vi "myRIO_BRig_Host_v0,21.vi"() -> ()   [LabVIEW 2014]
panel:
  out "graph":i32(graph)
  out "output_strAccum":string
  out "output_iTrial":i32
  out "BlockL_T2R_cur":u16 caption="Trials2Reward"
  out "BlockL_BTPR_cur":u16 caption="BadTrialsPostReward"
  out "BlockL_T2R_avg":dbl caption="Trials2Reward" format="%#_3g"
  out "BlockL_BTPR_avg":dbl caption="BadTrialsPostReward" format="%#_3g"
  out "BlockR_T2R_cur":u16 caption="Trials2Reward"
  out "BlockR_BTPR_cur":u16 caption="BadTrialsPostReward"
  out "BlockR_T2R_avg":dbl caption="Trials2Reward" format="%#_3g"
  out "BlockR_BTPR_avg":dbl caption="BadTrialsPostReward" format="%#_3g"
  out "RunTime_minutes":u16
  out "RunTime_seconds":u16
  out "error out 2":errorcluster caption="error out"
  in  "dataIn_maxTrialsDisplayed":u16 caption="Number of Trials Displayed\n( 0 = all trials )"
  in  "colorIn_timeout":u32(colorbox)=7468543 caption="Choice Timeout"
  in  "colorIn_wrong/cue":u32(colorbox)=16728618 caption="Wrong Choice or\nLicked During Cue"
  in  "colorIn_reward":u32(colorbox)=5898088 caption="Reward"
  in  "colorIn_unknown":u32(colorbox)=16449331 caption="Unknown Trial Status"
  in  "LoadPrevSettings":bool
  out "dataOut_plot":cluster{i32[], i32[]}[](graph)
  out "iBlock":u16
  out "iTrial":u16
  in  "stop":bool
  # "Exp Stats"
  # "Current Block Stats"
  # "Trials 2 Reward\n\nBad Trials\nPost Reward"
  # "Left Spout    Right Spout"
  # "Run Time\n\n   minutes    seconds"
  # "Average Block Stats"
  # "Trials 2 Reward\n\nBad Trials\nPost Reward"
  # "Left Spout    Right Spout"
  # "If you get ERROR 5 related to opening a file, press CONTINUE"
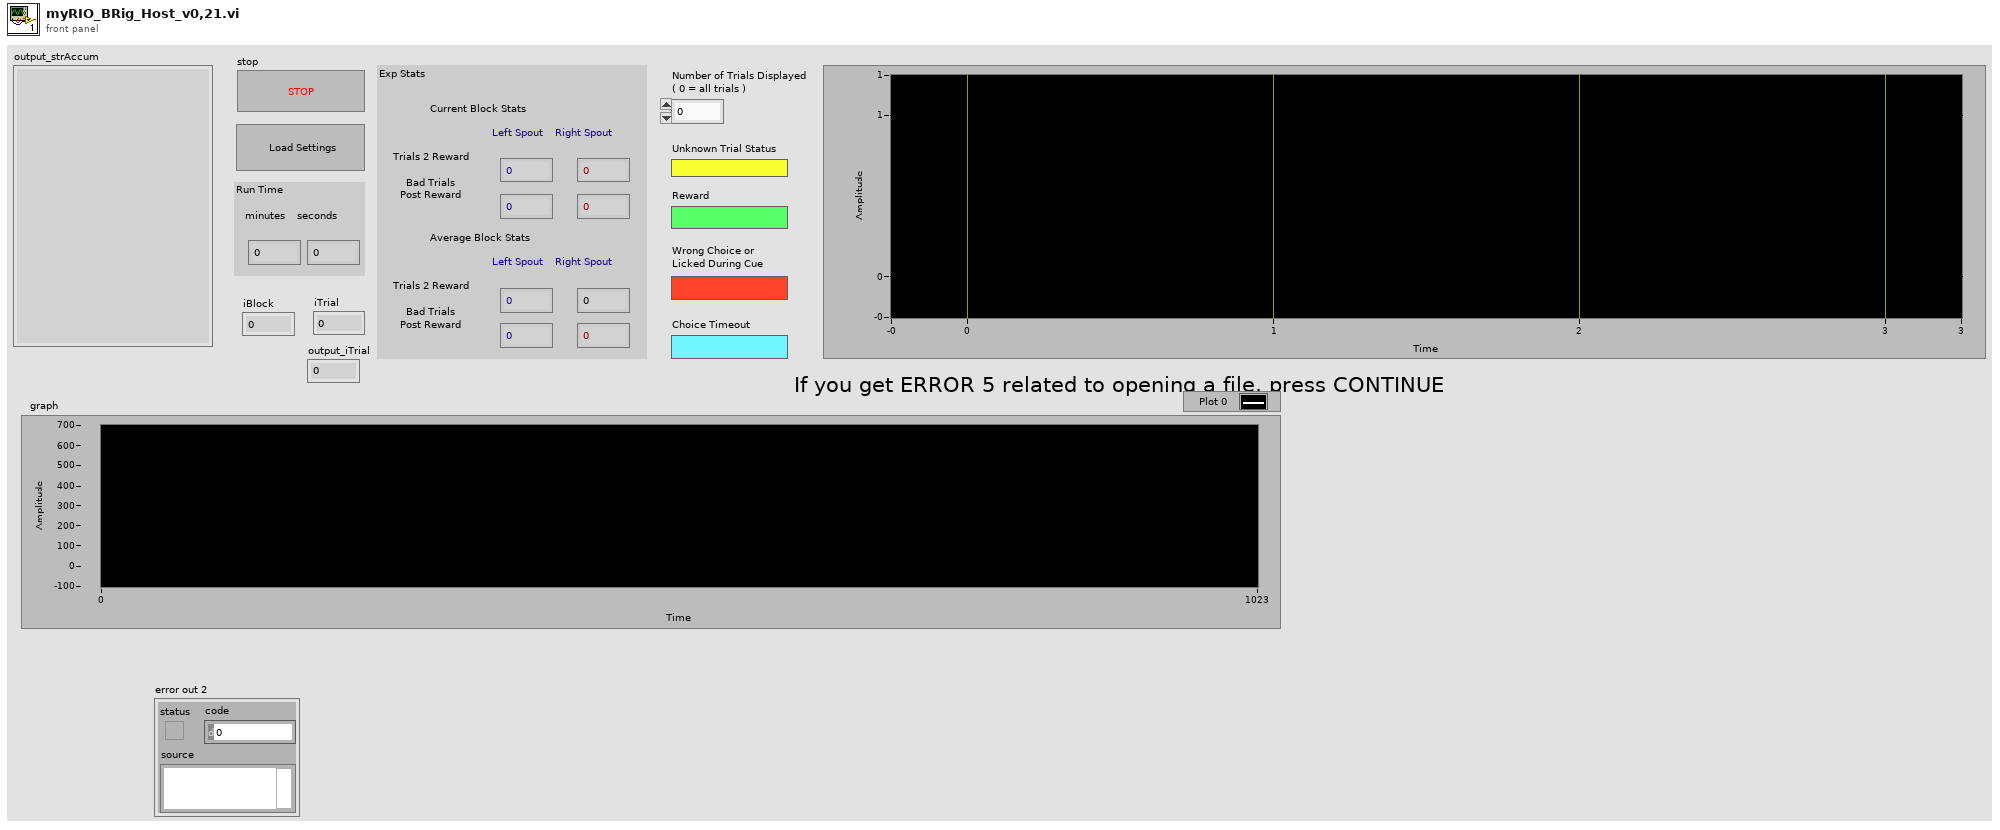
[diagram p1: front panel]
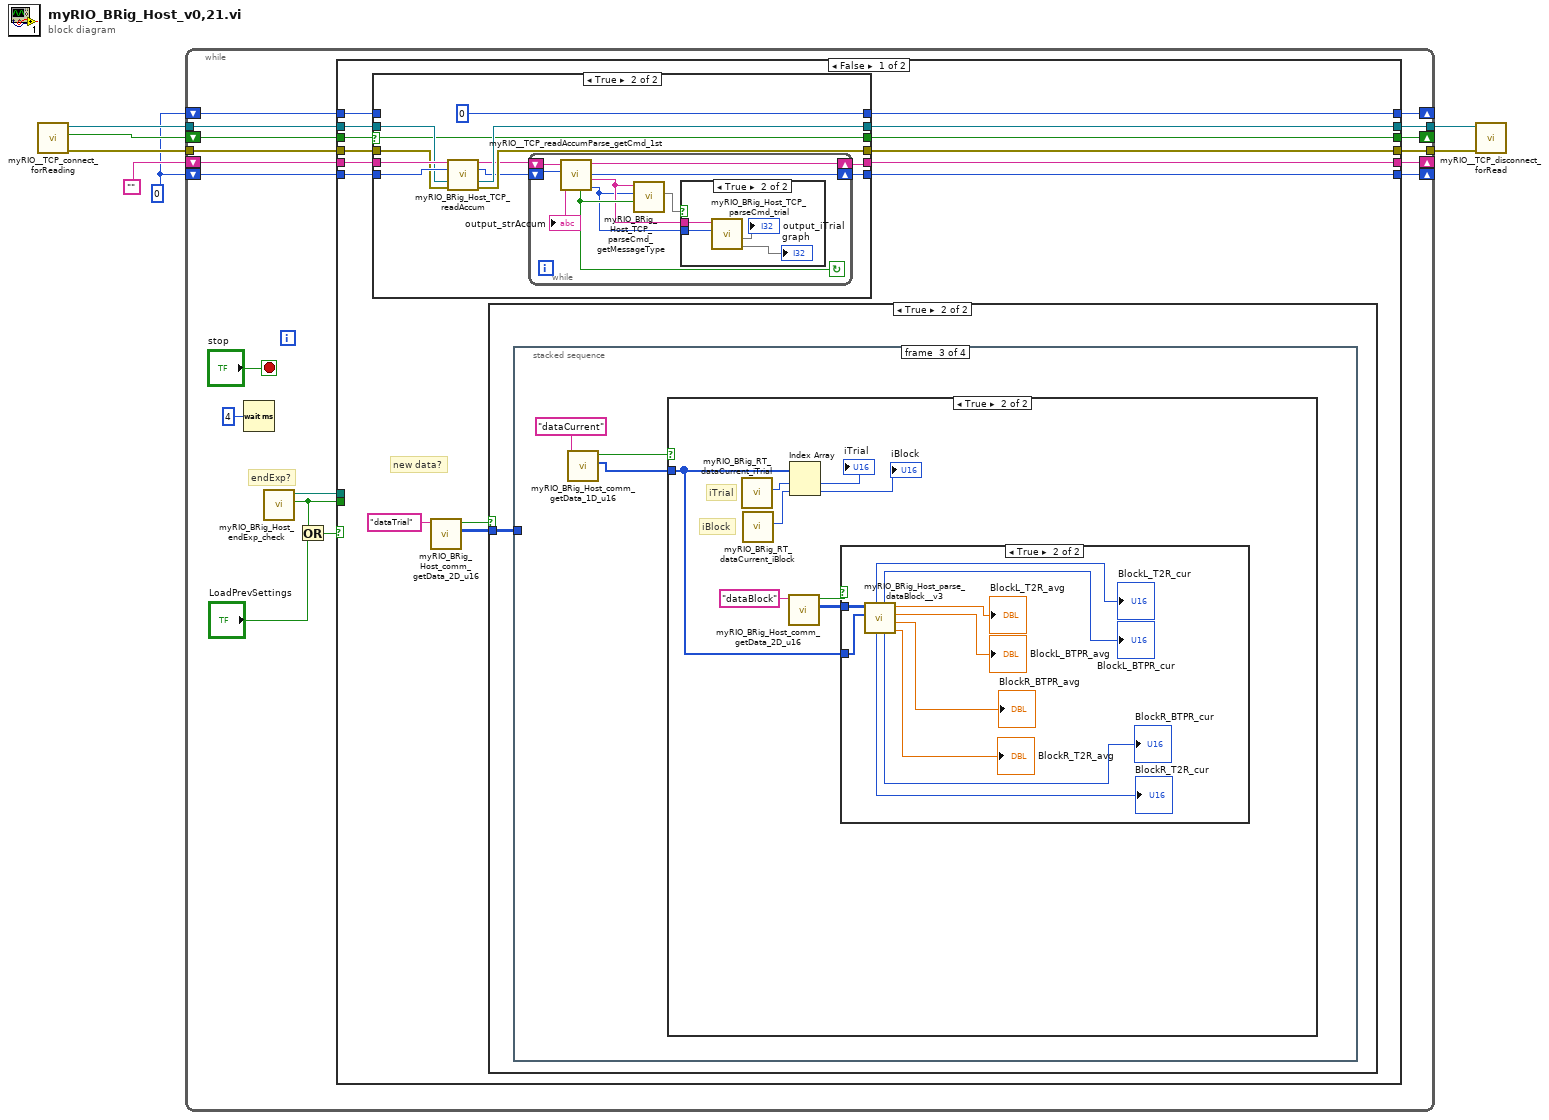
[diagram p0: block diagram]
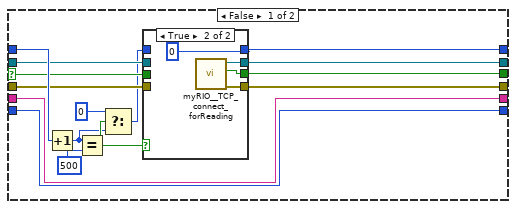
[diagram p2: hidden frame]
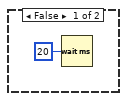
[diagram p5: hidden frame]
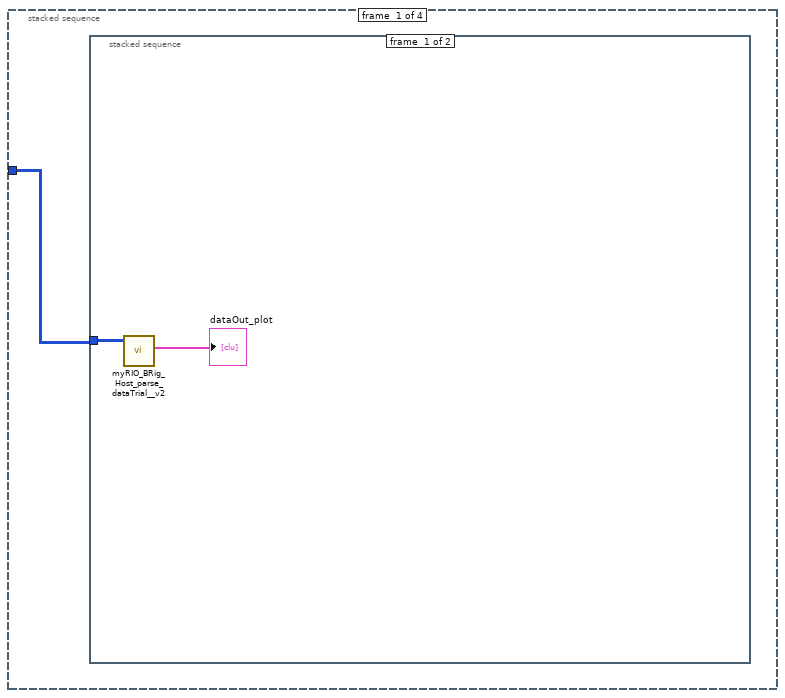
[diagram p6: hidden frame]
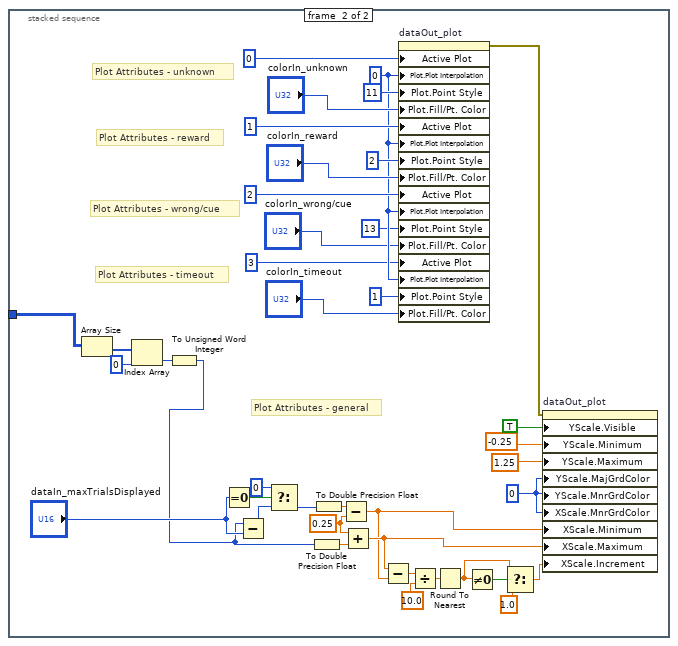
[diagram p7: hidden frame]
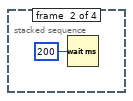
[diagram p8: hidden frame]
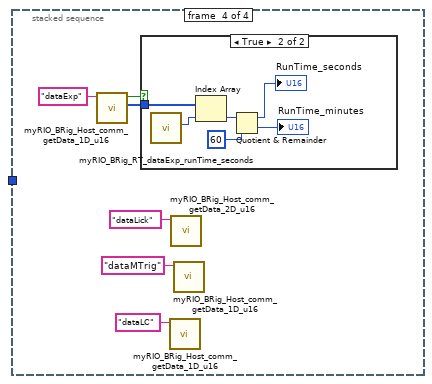
[diagram p11: hidden frame]
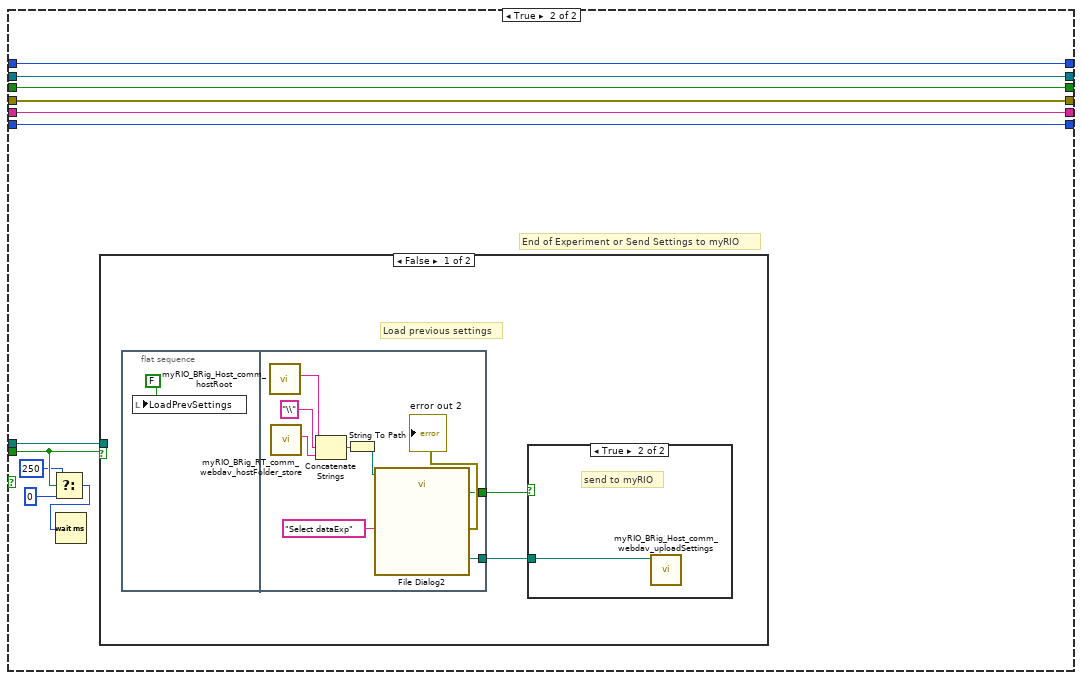
[diagram p13: hidden frame]
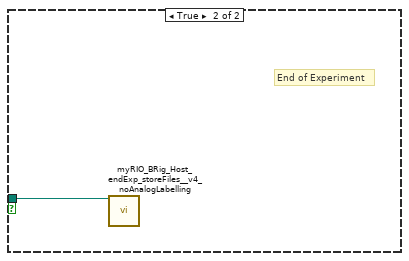
[diagram p15: hidden frame]
diagram:
  w1 = 0
  n1 = call "myRIO__TCP_connect_forReading.vi"() -> ("output_error"=w6:errorcluster, "output_connected"=w5:bool, "output_hTCP"=w7:refnum<k5>)  [unwired: 9 in]
  n2 = while {
    tunnel: w7 -> [w19]
    tunnel: w6 -> [w17]
    tunnel: [w18] -> w4
    tunnel: [w16] -> w3
    shift-right: [w13] -> _
    shift-left: "" -> [w15]
    shift-right: [w12] -> _
    shift-left: w1 -> [w14]
    shift-right: [w10] -> _
    shift-left: w5 -> [w11]
    shift-right: [w8] -> _
    shift-left: w1 -> [w9]
    stop <- "stop" stop-if-true
    # "endExp?"
    n3 = Wait (ms)(milliseconds to wait=u32 4) -> ()  [unwired: 1 out]
    n4 = call "myRIO_BRig_Host_endExp_check.vi"() -> ("output_IendExp"=w23:bool, "output_filePath_expExp"=w22:path)  [unwired: 10 in]
    n5 = Or(x=w23, y="LoadPrevSettings") -> (x .or. y?=w24:bool)
    n6 = case shown="False" w24 {
      tunnel: w23 -> [_ w176]
      tunnel: w22 -> [_ w177]
      tunnel: w19 -> [w33 w172]
      tunnel: [w32 w172] -> w18
      tunnel: w17 -> [w31 w171]
      tunnel: [w30 w171] -> w16
      tunnel: w15 -> [w37 w170]
      tunnel: w14 -> [w36 w169]
      tunnel: [w35 w170] -> w13
      tunnel: [w34 w169] -> w12
      tunnel: w11 -> [w29 w168]
      tunnel: [w28 w168] -> w10
      tunnel: w9 -> [w27 w167]
      tunnel: [w26 w167] -> w8
      frame False {
        # "new data?"
        n7 = case shown="True" w29 {
          selector: w29 -> [w48 w69]
          tunnel: w37 -> [w41 w75]
          tunnel: w36 -> [w42 w74]
          tunnel: [w41 w65] -> w35
          tunnel: [w42 w64] -> w34
          tunnel: w33 -> [w49 w73]
          tunnel: [w52 w72] -> w32
          tunnel: w31 -> [w47 w71]
          tunnel: [w51 w70] -> w30
          tunnel: [w50 w69] -> w28
          tunnel: w27 -> [w54 _]
          tunnel: [w53 0] -> w26
          frame False {
            n8 = Increment(x=w54) -> (x+1=w45:i32)
            n9 = Equal?(x=w45, y=500) -> (x = y?=w46:bool)
            n10 = Select(t=0, s=w46, f=w45) -> (s? t:f=w43:i32)
            n11 = case shown="True" w46 {
              tunnel: w43 -> [w59 _]
              tunnel: [w59 0] -> w53
              tunnel: [w58 w62] -> w52
              tunnel: [w56 w61] -> w51
              tunnel: [w57 w60] -> w50
              tunnel: w49 -> [w58 _]
              tunnel: w48 -> [w57 _]
              tunnel: w47 -> [w56 _]
              frame False {
              }
              frame True {
                n12 = call "myRIO__TCP_connect_forReading.vi"() -> ("output_error"=w61:errorcluster, "output_connected"=w60:bool, "output_hTCP"=w62:refnum<k5>)  [unwired: 9 in]
              }
            }
          }
          frame True {
            n13 = call "myRIO_BRig_Host_TCP_readAccum.vi"("input_strAccum"=w75, "input_count"=w74, "input_handle_TCP"=w73, "input_error"=w71) -> ("output_strAccum"=w67:string, "output_count"=w66:i32, "output_handle_TCP"=w72:refnum<k5>, "output_error"=w70:errorcluster)  [unwired: 8 in]
            n14 = while {
              shift-right: [w81] -> w65
              shift-left: w67 -> [w83]
              shift-right: [w80] -> w64
              shift-left: w66 -> [w82]
              stop <- w78 continue-if-true
              n15 = call "myRIO__TCP_readAccumParse_getCmd_1st.vi"("input_count"=w82, "input_strAccum"=w83) -> ("output_countCmd"=w76:i32, "output_strCmd"=w77:string, "output_count"=w80:i32, "output_strAccum"=w81:string, "output_haveCmd"=w78:bool)  [unwired: 5 in]
              "output_strAccum" <- w81
              n16 = call "myRIO_BRig_Host_TCP_parseCmd_getMessageType.vi"("input_haveCmd"=w78, "input_countCmd"=w76, "input_strCmd"=w77) -> (2:w79)  [unwired: 7 in, 1 out]
              n17 = case shown="True" w79 {
                tunnel: w77 -> [_ w87]
                tunnel: w76 -> [_ w86]
                frame False {
                }
                frame True {
                  n18 = call "myRIO_BRig_Host_TCP_parseCmd_trial.vi"("input_countCmd"=w86, "input_strCmd"=w87) -> (0:→"graph", 1:→"output_iTrial")  [unwired: 6 in, 2 out]
                }
              }
            }
          }
        }
        n19 = call "myRIO_BRig_Host_comm_getData_2D_u16.vi"("input_fileName"="dataTrial") -> ("output_data_2D"=w38:u16[][], "output_I_data"=w39:bool)  [unwired: 9 in]
        n20 = case shown="True" w39 {
          tunnel: w38 -> [_ w89]
          frame False {
            n21 = Wait (ms)(milliseconds to wait=u32 20) -> ()  [unwired: 1 out]
          }
          frame True {
            n22 = stacked-sequence {
              tunnel: w89 -> [w90 _ _ _]
              frame #0 {
                n23 = stacked-sequence {
                  tunnel: w90 -> [w91 w97]
                  frame #0 {
                    n24 = call "myRIO_BRig_Host_parse_dataTrial__v2.vi"("arrayIn_dataTrial"=w91) -> ("appended array"=→"dataOut_plot":cluster{i32[], i32[]}[])  [unwired: 10 in]
                  }
                  frame #1 {
                    w112 = 0.25 ("y")
                    w116 = u32 0 ("Y Scale.Grid Colors:Major Color")
                    w125 = u8 0 ("Plot.Plot Interpolation")
                    # "Plot Attributes - general"
                    # "Plot Attributes - timeout"
                    # "Plot Attributes - wrong/cue"
                    # "Plot Attributes - reward"
                    # "Plot Attributes - unknown"
                    n25 = Array Size(array=w97) -> (size(s)=w99:i32[])
                    n26 = Index Array(array=w99, index=0) -> (element=w95:i32)
                    n27 = To Unsigned Word Integer(number=w95) -> (unsigned 16bit integer=w94:u16)
                    n28 = Equal To 0?(x="dataIn_maxTrialsDisplayed") -> (x = 0?=w115:bool)
                    n29 = Subtract(x=w94, y="dataIn_maxTrialsDisplayed") -> (x-y=w114:u16)
                    n30 = Select(t=u16 0, s=w115, f=w114) -> (s? t:f=w109:u16)
                    n31 = To Double Precision Float(number=w94) -> (double precision float=w111:dbl)
                    n32 = To Double Precision Float(number=w109) -> (double precision float=w110:dbl)
                    n33 = Subtract(x=w110, y=w112) -> (x-y=w101:dbl)
                    n34 = Add(x=w112, y=w111) -> (x+y=w102:dbl)
                    n35 = Subtract(x=w102, y=w101) -> (x-y=w108:dbl)
                    n36 = property on="dataOut_plot" class="XYGraph (strict)"("Active Plot"=u32 0, "Plot.Plot Interpolation"=w125, "Plot.Point Style"=u8 11, "Plot.Fill/Pt. Color"="colorIn_unknown", "Active Plot"=u32 1, "Plot.Plot Interpolation"=w125, "Plot.Point Style"=u8 2, "Plot.Fill/Pt. Color"="colorIn_reward", "Active Plot"=u32 2, "Plot.Plot Interpolation"=w125, "Plot.Point Style"=u8 13, "Plot.Fill/Pt. Color"="colorIn_wrong/cue", "Active Plot"=u32 3, "Plot.Plot Interpolation"=w125, "Plot.Point Style"=u8 1, "Plot.Fill/Pt. Color"="colorIn_timeout") -> (error out=w100:errorcluster)  [unwired: 2 in, 1 out]
                    n37 = Divide(x=w108, y=10.0) -> (x/y=w106:dbl)
                    n38 = Round To Nearest(number=w106) -> (nearest integer value=w104:dbl)
                    n39 = Not Equal To 0?(x=w104) -> (x != 0?=w105:bool)
                    n40 = Select(t=w104, s=w105, f=1.0) -> (s? t:f=w103:dbl)
                    n41 = property on="dataOut_plot" class="XYGraph (strict)"(error in=w100, "YScale.Visible"=TRUE ("Y Scale.Visible"), "YScale.Minimum"=-0.25 ("Y Scale.Range:Minimum"), "YScale.Maximum"=1.25 ("Y Scale.Range:Maximum"), "YScale.MajGrdColor"=w116, "YScale.MnrGrdColor"=w116, "XScale.MnrGrdColor"=w116, "XScale.Minimum"=w101, "XScale.Maximum"=w102, "XScale.Increment"=w103) -> ()  [unwired: 1 in, 2 out]
                  }
                }
              }
              frame #1 {
                n42 = Wait (ms)(milliseconds to wait=u32 200) -> ()  [unwired: 1 out]
              }
              frame #2 {
                n43 = call "myRIO_BRig_Host_comm_getData_1D_u16.vi"("input_fileName"="dataCurrent") -> ("output_data_1D"=w134:u16[], "output_I_data"=w135:bool)  [unwired: 9 in]
                n44 = case shown="True" w135 {
                  tunnel: w134 -> [_ w137]
                  frame False {
                  }
                  frame True {
                    # "iBlock"
                    # "iTrial"
                    n45 = call "myRIO_BRig_RT_dataCurrent_iTrial.vi"() -> ("output_iTrial"=w144:i32)  [unwired: 11 in]
                    n46 = call "myRIO_BRig_RT_dataCurrent_iBlock.vi"() -> ("output_iBlock"=w143:i32)  [unwired: 11 in]
                    n47 = call "myRIO_BRig_Host_comm_getData_2D_u16.vi"("input_fileName"="dataBlock") -> ("output_data_2D"=w138:u16[][], "output_I_data"=w139:bool)  [unwired: 9 in]
                    n48 = Index Array(array=w137, index #1=w144, index #2=w143) -> (element #1=→"iTrial":u16, element #2=→"iBlock":u16)
                    n49 = case shown="True" w139 {
                      tunnel: w138 -> [_ w146]
                      tunnel: w137 -> [_ w145]
                      frame False {
                      }
                      frame True {
                        n50 = call "myRIO_BRig_Host_parse_dataBlock__v3.vi"("input_dataCurrent"=w145, "input_dataBlock"=w146) -> ("BlockR_T2R_avg"=→"BlockR_T2R_avg":dbl, "BlockR_BTPR_avg"=→"BlockR_BTPR_avg":dbl, "BlockL_BTPR_avg"=→"BlockL_BTPR_avg":dbl, "BlockL_T2R_avg"=→"BlockL_T2R_avg":dbl, "BlockR_BTPR_cur"=→"BlockR_BTPR_cur":u16, "BlockL_BTPR_cur"=→"BlockL_BTPR_cur":u16, "BlockR_T2R_cur"=→"BlockR_T2R_cur":u16, "BlockL_T2R_cur"=→"BlockL_T2R_cur":u16)  [unwired: 2 in]
                      }
                    }
                  }
                }
              }
              frame #3 {
                n51 = call "myRIO_BRig_Host_comm_getData_1D_u16.vi"("input_fileName"="dataExp") -> ("output_data_1D"=w158:u16[], "output_I_data"=w159:bool)  [unwired: 9 in]
                n52 = case shown="True" w159 {
                  tunnel: w158 -> [_ w166]
                  frame False {
                  }
                  frame True {
                    n53 = call "myRIO_BRig_RT_dataExp_runTime_seconds.vi"() -> ("output_RunTime_minutes"=w165:i32)  [unwired: 11 in]
                    n54 = Index Array(array=w166, index=w165) -> (element=w164:u16)
                    n55 = Quotient & Remainder(x=w164, y=u16 60) -> (x-y*floor(x/y)=→"RunTime_seconds":u16, floor(x/y)=→"RunTime_minutes":u16)
                  }
                }
                n56 = call "myRIO_BRig_Host_comm_getData_1D_u16.vi"("input_fileName"="dataLC") -> ()  [unwired: 9 in, 2 out]
                n57 = call "myRIO_BRig_Host_comm_getData_2D_u16.vi"("input_fileName"="dataLick") -> ()  [unwired: 9 in, 2 out]
                n58 = call "myRIO_BRig_Host_comm_getData_1D_u16.vi"("input_fileName"="dataMTrig") -> ()  [unwired: 9 in, 2 out]
              }
            }
          }
        }
      }
      frame True {
        # "End of Experiment or Send Settings to myRIO"
        n59 = Select(t=u32 250 ("milliseconds to wait"), s=w176, f=u32 0 ("milliseconds to wait")) -> (s? t:f=w174:u32)
        n60 = Wait (ms)(milliseconds to wait=w174) -> ()  [unwired: 1 out]
        n61 = case shown="False" w176 {
          tunnel: w177 -> [_ w191]
          frame False {
            # "Load previous settings"
            n62 = flat-sequence {
              tunnel: [w183] -> w178
              tunnel: [w182] -> w179
              frame #0 {
                n63 = local write "LoadPrevSettings"(FALSE ("LoadPrevSettings")) -> ()
              }
              frame #1 {
                n64 = call "myRIO_BRig_Host_comm_hostRoot.vi"() -> ("output_hostRoot"=w185:string)  [unwired: 11 in]
                n65 = call "myRIO_BRig_RT_comm_webdav_hostFolder_store.vi"() -> ("output_HostFolder"=w187:string)  [unwired: 11 in]
                n66 = Concatenate Strings(w185, "\\" ("string"), w187) -> (w189:string)
                n67 = String To Path(string=w189) -> (path=w188:path)
                n68 = call "File Dialog2"("start path"=w188, "prompt"="Select dataExp") -> ("selected path"=w183:path, "exists"=w182:bool, "error out"=→"error out 2":errorcluster)  [unwired: 10 in, 1 out]
              }
            }
            n69 = case shown="True" w179 {
              tunnel: w178 -> [_ w180]
              frame False {
                # "invalid file\nor\ncancelled"
              }
              frame True {
                # "send to myRIO"
                n70 = call "myRIO_BRig_Host_comm_webdav_uploadSettings.vi"("input_filePath"=w180) -> ()  [unwired: 11 in]
              }
            }
          }
          frame True {
            # "End of Experiment"
            n71 = call "myRIO_BRig_Host_endExp_storeFiles__v4_noAnalogLabelling.vi"("input_filePath"=w191) -> ()  [unwired: 15 in]
          }
        }
      }
    }
  }
  n72 = call "myRIO__TCP_disconnect_forRead.vi"("input_error"=w3, "input_hTCP"=w4) -> ()  [unwired: 9 in, 1 out]
